vi "sub_Sync_Receiver.vi"(6 "filter parameters":T2={"Alpha"=0.5, "Filter Length"=6, "TX Filter"=enum."Root Raised Cos"} {"Alpha" format="%.2f"}, 7 "Packet Parameters in":T1={"Length of sync sequence (50)"=50, "Number of message bits"=128, "Number of guardbits"=40, "Sync PN sequence order (31)"=31, "Number of header bits"=16, "Packet Pad [samples]"=0}, 8 "error in (no error)":errorcluster, 9 "QPSK System Parameters":T3={"Samples per Symbol"=8, "symbol map"=[], "Differential PSK"=enum."disable", "PSK type"=0, "M-PSK"=4} {"PSK type" items=["normal", "shifted", "offset"]; "symbol map" format="%.3f"}, 10 "Rx Parameters":T4={"Rx IQ Sampling\nRate [s/sec]"=400000.0, "Rx\nFrequency [Hz]"=5795000000.0, "Rx Gain [dB]"=20.0, "Rx Antenna"="RX1"} {"Rx Gain [dB]" format="%#.6p"; "Rx\nFrequency [Hz]" format="%#.6p"; "Rx IQ Sampling\nRate [s/sec]" format="%#.6p"}, 11 "session handle":refnum<k15>) -> (0 "error out":errorcluster, 3 "session handle out":refnum<k15>)   [LabVIEW 2014]
uses:
  <instrlib>/niUSRP/niUSRP Fetch Rx Data (CDB Cluster).vi
panel:
  in  "Sync index tolerance":i32=10
  out "Iterations":i32
  out "Expected Xcorr Index":i32
  out "Sync Correct?":bool
  out "Sync Stable?":bool
  out "Now Max Xcorr Index":i32
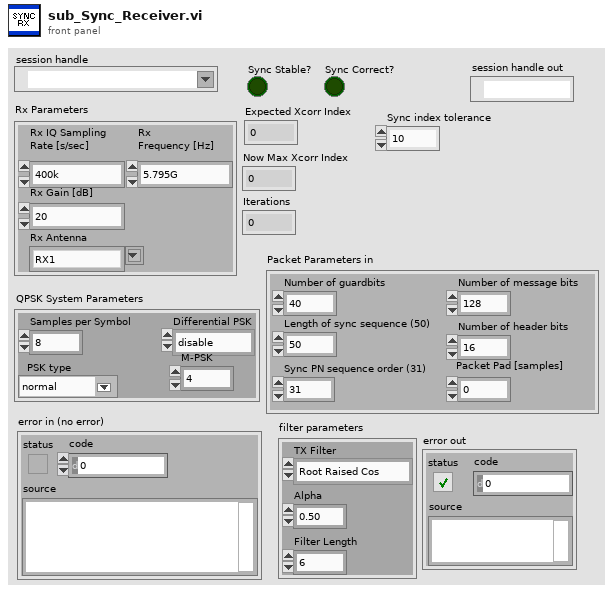
[diagram p1: front panel]
types:
  T1 = cluster{"Length of sync sequence (50)":i32, "Number of message bits":i32, "Number of guardbits":i32, "Sync PN sequence order (31)":i32, "Number of header bits":i32, "Packet Pad [samples]":i32}
  T2 = cluster{"Alpha":dbl, "Filter Length":i32, "TX Filter":enum16{"none", "Raised Cosine", "Root Raised Cos", "Gaussian"}}
  T3 = cluster{"Samples per Symbol":i32, "symbol map":cdb[], "Differential PSK":enum16{"disable", "enable"}, "PSK type":u16, "M-PSK":i32}
  T4 = cluster{"Rx IQ Sampling\nRate [s/sec]":dbl, "Rx\nFrequency [Hz]":dbl, "Rx Gain [dB]":dbl, "Rx Antenna":string}
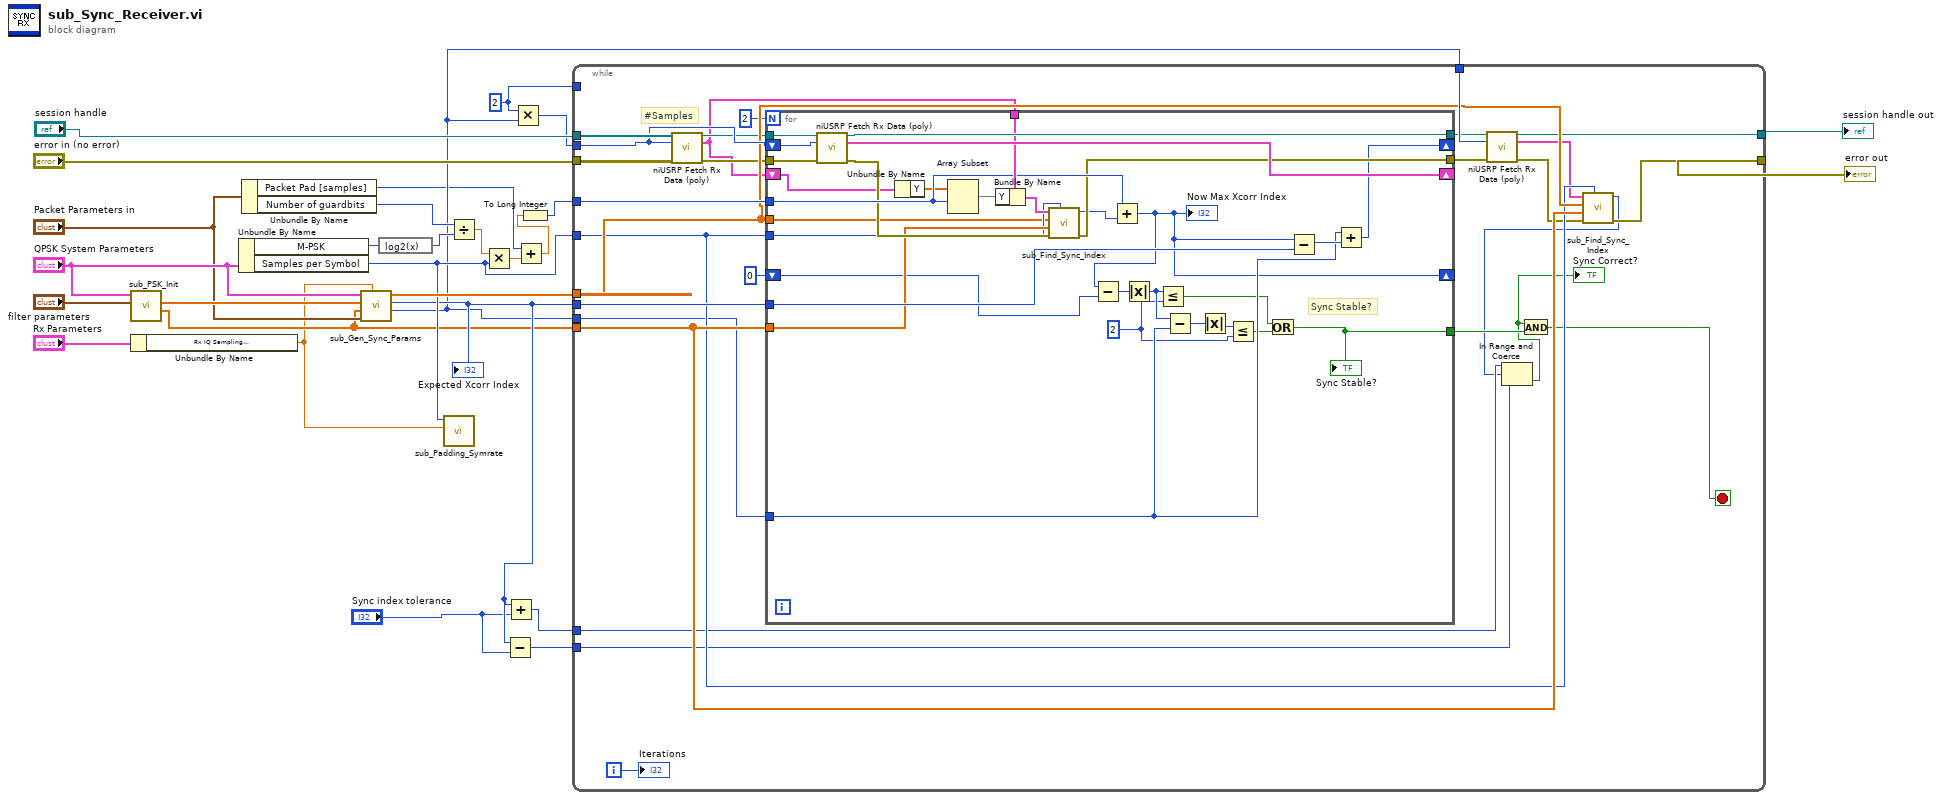
[diagram p0: block diagram]
diagram:
  w7 = 2 ("x")
  n1 = call "sub_PSK_Init.vi"("filter parameters in"="filter parameters", "QPSK System Parameters in"="QPSK System Parameters") -> ("matched filter coefficients"=w5:dbl[], "pulse shaping filter coefficients"=w25:dbl[])  [unwired: 7 in, 1 out]
  n2 = Unbundle By Name("Rx Parameters") -> ("Rx IQ Sampling\nRate [s/sec]"=w4:dbl)
  n3 = Unbundle By Name("QPSK System Parameters") -> ("M-PSK"=w19:i32, "Samples per Symbol"=w12:i32)
  n4 = Unbundle By Name("Packet Parameters in") -> ("Packet Pad [samples]"=w2:i32, "Number of guardbits"=w23:i32)
  n5 = call "sub_Gen_Sync_Params.vi"("IQ Sampling\nRate [s/sec]"=w4, "Packet Parameters in"="Packet Parameters in", "matched filter coefficients"=w5, "pulse shaping filter coefficients"=w25, "QPSK System Parameters in"="QPSK System Parameters") -> ("Frame Length (samples)"=w3:i32, "Expected Xcorr Index"=w11:i32, "Sync Sequence Waveform"=w17:cdb[])  [unwired: 3 in, 1 out]
  "Expected Xcorr Index" <- w11
  n6 = expression code="log2(x)"(w19) -> (w18:i32)
  n7 = call "sub_Padding_Symrate.vi"("Tx IQ Sampling\nRate [s/sec]"=w4, "Samples per Symbol"=w12) -> ()  [unwired: 8 in, 2 out]
  n8 = Divide(x=w23, y=w18) -> (x/y=w22:dbl)
  n9 = Multiply(x=w22, y=w12) -> (x*y=w21:dbl)
  n10 = Subtract(x=w11, y="Sync index tolerance") -> (x-y=w8:i32)
  n11 = Add(x=w11, y="Sync index tolerance") -> (x+y=w9:i32)
  n12 = Multiply(x=w7, y=w3) -> (x*y=w13:i32)
  n13 = Add(x=w2, y=w21) -> (x+y=w16:dbl)
  n14 = To Long Integer(number=w16) -> (32bit integer=w1:i32)
  n15 = while {
    tunnel: "session handle" -> [w55]
    tunnel: "error in (no error)" -> [w54]
    tunnel: w13 -> [w53]
    tunnel: w1 -> [w56]
    tunnel: w17 -> [w50]
    tunnel: w5 -> [w49]
    tunnel: w12 -> [w47]
    tunnel: w11 -> [w52]
    tunnel: [w48] -> w15
    tunnel: [w46] -> w14
    tunnel: w3 -> [w51]
    tunnel: w9 -> [w44]
    tunnel: w8 -> [w43]
    tunnel: w7 -> [_]
    tunnel: w3 -> [w29]
    i -> [w45]
    stop <- w30 stop-if-true
    # "#Samples"
    n16 = call-poly <instrlib>:"niUSRP Fetch Rx Data (poly).vi"("session handle"=w55, "number of samples"=w53, "error in (no error)"=w54) -> ("session handle out"=w41:refnum<k15>, "data"=w34:cluster{"t0":dbl, "dt":dbl, "Y":cdb[]}, "error out"=w40:errorcluster)  [unwired: 9 in, 1 out]
    n17 = for {
      N: 2 ("index") -> [_]
      tunnel: w41 -> [w87]
      tunnel: w40 -> [w86]
      shift-right: [w83] -> _
      shift-left: w34 -> [w63]
      tunnel: w56 -> [w78]
      tunnel: w50 -> [w57]
      tunnel: w49 -> [w74]
      tunnel: w47 -> [w73]
      shift-right: [w58] -> _
      shift-left: w53 -> [w85]
      shift-right: [w59] -> _
      shift-left: 0 -> [w72]
      tunnel: w29 -> [w70]
      tunnel: w52 -> [w82]
      tunnel: [w81] -> w39
      tunnel: [w80] -> w37
      tunnel: [w77] -> w36
      tunnel: w34 -> [w79]
      w66 = 2 ("y")
      # "Sync Stable?"
      n18 = call-poly <instrlib>:"niUSRP Fetch Rx Data (poly).vi"("session handle"=w87, "number of samples"=w85, "error in (no error)"=w86) -> ("session handle out"=w80:refnum<k15>, "data"=w83:cluster{"t0":dbl, "dt":dbl, "Y":cdb[]}, "error out"=w76:errorcluster)  [unwired: 9 in, 1 out]
      n19 = Unbundle By Name(w63) -> ("Y"=w61:cdb[])
      n20 = Array Subset(array=w61, index=w78) -> (w60:cdb[])  [unwired: 1 in]
      n21 = Bundle By Name(cluster=w79, "Y"=w60) -> (w84:cluster{"t0":dbl, "dt":dbl, "Y":cdb[]})
      n22 = call "sub_Find_Sync_Index.vi"("samples per symbol (16)"=w73, "error in (no error)"=w76, "matched filter coefficients"=w74, "Sync Sequence Waveform"=w57, "Input Complex Waveform"=w84) -> ("error out"=w77:errorcluster, "Max Xcorr Index"=w62:i32)  [unwired: 4 in, 1 out]
      n23 = Add(x=w78, y=w62) -> (x+y=w59:i32)
      "Now Max Xcorr Index" <- w59
      n24 = Subtract(x=w59, y=w72) -> (x-y=w71:i32)
      n25 = Absolute Value(x=w71) -> (abs(x)=w69:i32)
      n26 = Less Or Equal?(x=w69, y=w66) -> (x <= y?=w64:bool)
      n27 = Subtract(x=w69, y=w70) -> (x-y=w68:i32)
      n28 = Absolute Value(x=w68) -> (abs(x)=w67:i32)
      n29 = Less Or Equal?(x=w67, y=w66) -> (x <= y?=w65:bool)
      n30 = Or(x=w64, y=w65) -> (x .or. y?=w81:bool)
      "Sync Stable?" <- w81
      n31 = Subtract(x=w59, y=w82) -> (x-y=w75:i32)
      n32 = Add(x=w70, y=w75) -> (x+y=w58:i32)
    }
    n33 = call-poly <instrlib>:"niUSRP Fetch Rx Data (poly).vi"("session handle"=w37, "number of samples"=w51, "error in (no error)"=w36) -> ("session handle out"=w48:refnum<k15>, "data"=w35:cluster{"t0":dbl, "dt":dbl, "Y":cdb[]}, "error out"=w33:errorcluster)  [unwired: 9 in, 1 out]
    n34 = call "sub_Find_Sync_Index.vi"("samples per symbol (16)"=w47, "error in (no error)"=w33, "matched filter coefficients"=w49, "Sync Sequence Waveform"=w50, "Input Complex Waveform"=w35) -> ("error out"=w46:errorcluster, "Max Xcorr Index"=w32:i32)  [unwired: 4 in, 1 out]
    n35 = In Range and Coerce(upper limit=w44, x=w32, lower limit=w43) -> (In Range?=w31:bool)  [unwired: 1 out]
    "Sync Correct?" <- w31
    n36 = And(x=w31, y=w39) -> (x .and. y?=w30:bool)
    "Iterations" <- w45
  }
  "session handle out" <- w15
  "error out" <- w14
